vi "cdex_unwrap signal.vi"(1 "initialize":bool, 2 "input":dbl format="%0.2f", 4 "wrap range":dbl=6.283185307179586) -> (7 "output":dbl format="%0.2f")   [LabVIEW 2009]
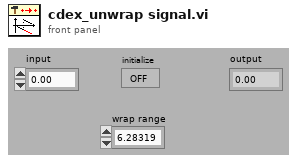
[diagram p1: front panel]
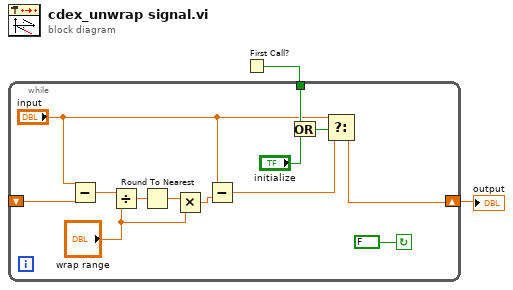
[diagram p0: block diagram]
diagram:
  n1 = First Call?() -> (First Call?: T/F=w2:bool)
  n2 = while {
    tunnel: w2 -> [w11]
    shift-left: _ -> [w14]
    shift-right: [w15] -> w1
    stop <- FALSE continue-if-true
    n3 = Subtract(x="input", y=w14) -> (x-y=w4:dbl)
    n4 = Divide(x=w4, y="wrap range") -> (x/y=w9:dbl)
    n5 = Round To Nearest(number=w9) -> (nearest integer value=w8:dbl)
    n6 = Multiply(x=w8, y="wrap range") -> (x*y=w3:dbl)
    n7 = Subtract(x="input", y=w3) -> (x-y=w5:dbl)
    n8 = Or(x=w11, y="initialize") -> (x .or. y?=w10:bool)
    n9 = Select(t="input", s=w10, f=w5) -> (s? t:f=w15:dbl)
  }
  "output" <- w1
